vi "Initialize EtherCAT youBot Wheel Motor.vi"(8 "error in (no error)":errorcluster, 11 "motor slave info in":T1 {"nodeAddr" format="%.0x"}) -> (0 "error out":errorcluster, 3 "KUKA youBot wheel motor_EtherCAT out":refnum<class "NI_Robotics_KUKA youBot Wheel Motor_EtherCAT.lvclass">)   [LabVIEW 2017, in "NI_Robotics_KUKA youBot Host.lvlib" / "NI_Robotics_KUKA youBot Wheel Motor_EtherCAT.lvclass"]
uses:
  <vilib>/robotics/KUKA youBot/Motor/Wheel Motor EtherCAT/NI_Robotics_KUKA youBot Wheel Motor_EtherCAT.lvclass
  <vilib>/robotics/KUKA youBot/EtherCAT/Motor Slave Info.ctl
  <vilib>/robotics/KUKA youBot/EtherCAT/LowLevel/Mater Handler.ctl
  <vilib>/robotics/KUKA youBot/EtherCAT/EtherCAT Command.ctl
  <vilib>/robotics/KUKA youBot/EtherCAT/CmdCtrls/Param Cmd.ctl
  <vilib>/robotics/KUKA youBot/Motor/Wheel Motor EtherCAT/NI_Robotics_KUKA youBot Wheel Motor_EtherCAT.lvclass/NI_Robotics_KUKA youBot Wheel Motor_EtherCAT.ctl
  <vilib>/robotics/KUKA youBot/NI_Robotics_KUKA youBot Host.lvlib
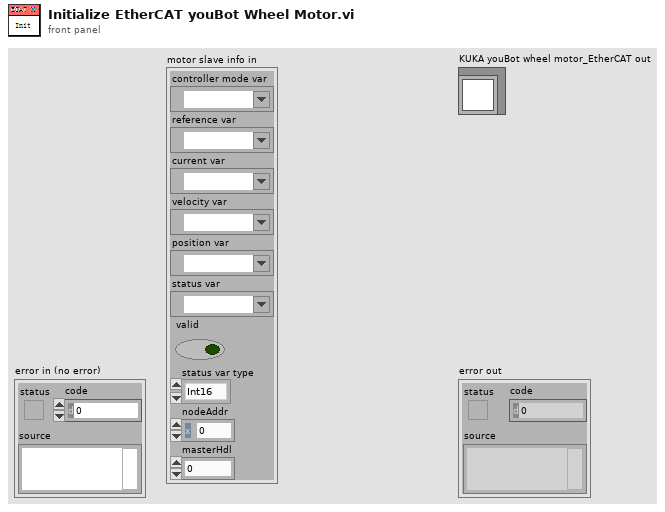
[diagram p1: front panel]
types:
  T1 = typedef "NI_Robotics_KUKA youBot Host.lvlib/Motor Slave Info.ctl" = cluster{"controller mode var":refnum<k21>, "reference var":refnum<k21>, "current var":refnum<k21>, "velocity var":refnum<k21>, "position var":refnum<k21>, "status var":refnum<k21>, "valid":bool, "status var type":enum16{"Int16", "Int32"}, "nodeAddr":u16, "masterHdl":T2}
  T2 = typedef "NI_Robotics_KUKA youBot Host.lvlib/Mater Handler.ctl" = i32
  T3 = typedef "NI_Robotics_KUKA youBot Host.lvlib/EtherCAT Command.ctl" = cluster{"Module":u8, "Cmd":T4, "Type":u8, "Bank":u8, "Val":u32}
  T4 = typedef "NI_Robotics_KUKA youBot Host.lvlib/Param Cmd.ctl" = u8
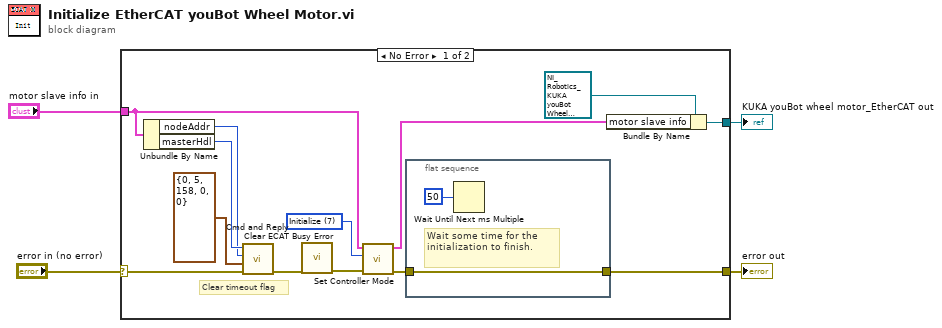
[diagram p0: block diagram]
diagram:
  n1 = case shown="No Error" "error in (no error)" {
    selector: "error in (no error)" -> [w10 w20]
    tunnel: [w12 w20] -> w1
    tunnel: [w17 _] -> w2
    tunnel: "motor slave info in" -> [w13 _]
    frame No Error {
      w16 = u8 7 items=["Motor Stop", "Positioning-Mode", "Velocity-Mode", "no more action", "set position to reference", "PWM-Mode", "Current-Mode", "Initialize"] ("controller mode")
      # "Clear timeout flag"
      n2 = Unbundle By Name(w13) -> ("nodeAddr"=w8:u16, "masterHdl"=w9:T2)
      n3 = call <vilib>:"Cmd and Reply.vi"("error in (no error)"=w10, "EtherCAT command"=T3 {"Module"=0, "Cmd"=5, "Type"=158, "Bank"=0, "Val"=0}, "nodeAddr in"=w8, "masterHdl in"=w9) -> ("error out"=w6:errorcluster)  [unwired: 3 in, 4 out]
      n4 = call <vilib>:"Clear ECAT Busy Error.vi"("error in (no error)"=w6) -> ("error out"=w5:errorcluster)  [unwired: 10 in]
      n5 = call <vilib>:"Set Controller Mode.vi"("error in (no error)"=w5, "controller mode"=w16, "motor slave info in"=w13) -> ("error out"=w11:errorcluster, "motor slave info out"=w14:T1)  [unwired: 6 in, 1 out]
      n6 = flat-sequence {
        tunnel: [w18] -> w12
        tunnel: w11 -> [w18]
        frame #0 {
          # "Wait some time for the initialization to finish."
          n7 = Wait Until Next ms Multiple(millisecond multiple=u32 50) -> ()  [unwired: 1 out]
        }
      }
      n8 = Bundle By Name(cluster=refnum<class "NI_Robotics_KUKA youBot Wheel Motor_EtherCAT.lvclass"> refnum ("NI_Robotics_KUKA youBot Host.lvlib:NI_Robotics_KUKA youBot Wheel Motor_EtherCAT.lvclass"), "motor slave info"=w14) -> (w17:refnum<class "NI_Robotics_KUKA youBot Wheel Motor_EtherCAT.lvclass">)
    }
    frame Error {
    }
  }
  "error out" <- w1
  "KUKA youBot wheel motor_EtherCAT out" <- w2
